vi "VP_to_ppm.vi"(11 "VP (Hgmm)":dbl) -> (3 "Saturated concentration (ppm)":dbl)   [LabVIEW 2016]
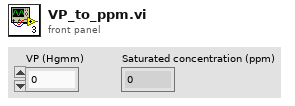
[diagram p1: front panel]
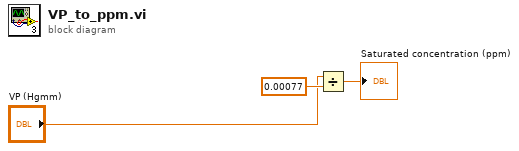
[diagram p0: block diagram]
diagram:
  n1 = Divide(x="VP (Hgmm)", y=0.00077) -> (x/y=→"Saturated concentration (ppm)":dbl)
